vi "外部交互全局.vi"() -> ()   [LabVIEW 2016]
panel:
  in  "当前瓶号":u16
  out "超标留样信号":bool
  in  "CODCr超标浓度":dbl
  in  "CODMn超标浓度":dbl
  in  "总氮超标浓度":dbl
  in  "总磷超标浓度":dbl
  in  "氨氮超标浓度":dbl
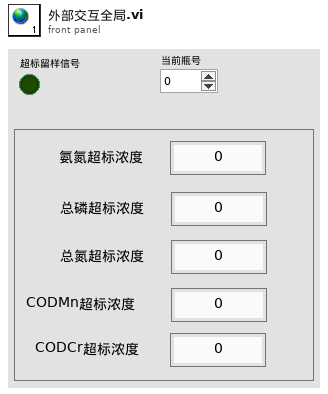
[diagram p1: front panel]
diagram:
